vi "Set Current Font.vi"(0 "report in":refnum<class "NI_report.lvclass">, 7 "font":T1, 11 "error in (no error)":errorcluster) -> (4 "report out":refnum<class "NI_report.lvclass">, 15 "error out":errorcluster)   [LabVIEW 2017, in "NI_ReportGenerationToolkit.lvlib"]
uses:
  <vilib>/addons/_office/NI_ReportGenerationToolkit.lvlib
  <vilib>/Utility/NIReport.llb/NI_report.lvclass
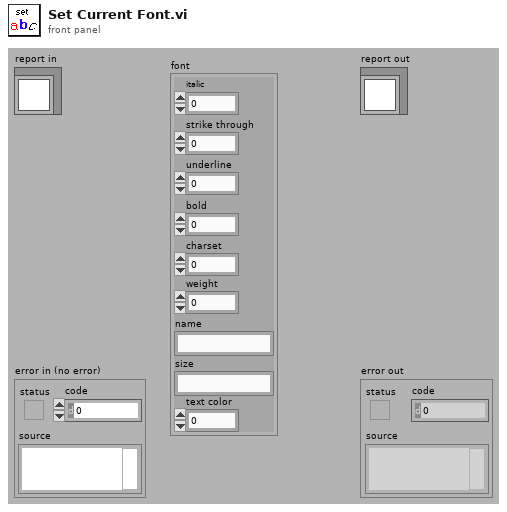
[diagram p1: front panel]
types:
  T1 = cluster{"italic":i32, "strike through":i32, "underline":i32, "bold":i32, "charset":i16, "weight":i16, "name":string, "size":string, "text color":u32}
  T2 = cluster{"Italic":enum16{"Italic Unchanged", "Italic On", "Italic Off"}, "Strike Through":enum16{"Strike Through Unchanged", "Strike Through On", "Strike Through Off"}, "Underline":enum16{"Underline Unchanged", "Underline On", "Underline Off"}, "Bold":enum16{"Bold Unchanged", "Bold On", "Bold Off"}}
  T3 = cluster{"Charset (-1)":i16, "Weight (-1)":i16, "Name":string, "Size":string}
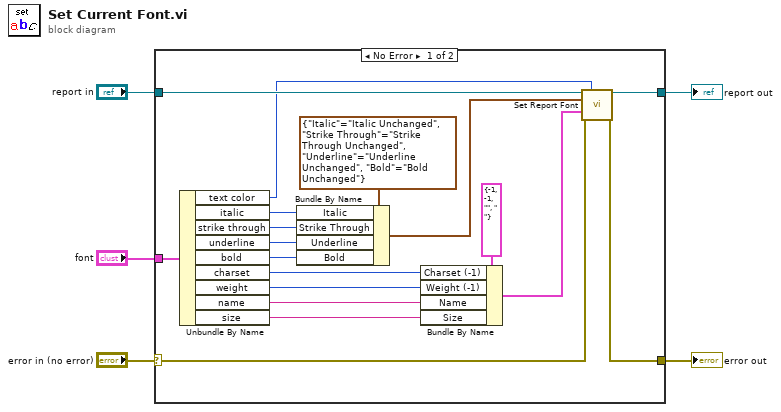
[diagram p0: block diagram]
diagram:
  n1 = case shown="No Error" "error in (no error)" {
    selector: "error in (no error)" -> [w8 w25]
    tunnel: [w7 w25] -> w4
    tunnel: [w9 w24] -> w2
    tunnel: "report in" -> [w10 w24]
    tunnel: "font" -> [w11 _]
    frame No Error {
      n2 = Unbundle By Name(w11) -> ("text color"=w6:u32, "italic"=w19:i32, "strike through"=w18:i32, "underline"=w17:i32, "bold"=w16:i32, "charset"=w15:i16, "weight"=w14:i16, "name"=w13:string, "size"=w12:string)
      n3 = Bundle By Name(cluster=T2 {"Italic"=enum."Italic Unchanged", "Strike Through"=enum."Strike Through Unchanged", "Underline"=enum."Underline Unchanged", "Bold"=enum."Bold Unchanged"} ("text options"), "Italic"=w19, "Strike Through"=w18, "Underline"=w17, "Bold"=w16) -> (w23:T2)
      n4 = Bundle By Name(cluster=T3 {"Charset (-1)"=-1, "Weight (-1)"=-1, "Name"="", "Size"=" "} ("font settings"), "Charset (-1)"=w15, "Weight (-1)"=w14, "Name"=w13, "Size"=w12) -> (w20:T3)
      n5 = call-dynamic "Set Report Font.vi"("report in"=w10, "text color (unchanged)"=w6, "text options"=w23, "font settings"=w20, "error in (no error)"=w8) -> ("report out"=w9:refnum<class "NI_report.lvclass">, "error out"=w7:errorcluster)  [unwired: 8 in, 1 out]
    }
    frame Error {
    }
  }
  "error out" <- w4
  "report out" <- w2
